vi "Task2InClass.vi"(10 "Numeric 2":dbl, 11 "Numeric":dbl) -> (3 "Numeric 3":dbl)   [LabVIEW 2016]
uses:
  <vilib>/express/express arith-compare/Formula/XNode/ExpressFormulaBlockNode.xnode
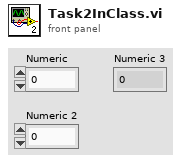
[diagram p1: front panel]
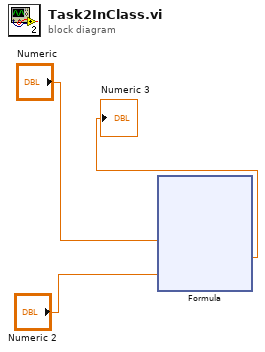
[diagram p0: block diagram]
diagram:
  n1 = xnode "Formula"("X1"="Numeric", "X2"="Numeric 2") -> ("Result"=→"Numeric 3":dbl)  [unwired: 1 in, 1 out]
